vi "read_GPX_file.vi"(4 "error in":errorcluster, 7 "GPX File Path":path) -> (0 "error out":errorcluster, 1 "position Graph":cluster{"X":dbl, "Y":dbl}[](graph), 2 "lat/lon position":cluster{timestamp[], dbl[], dbl[]}, 3 "XY Speed data":cluster{timestamp[], dbl[]})   [LabVIEW 2020]
panel:
  out "trk.trkseg data":T1
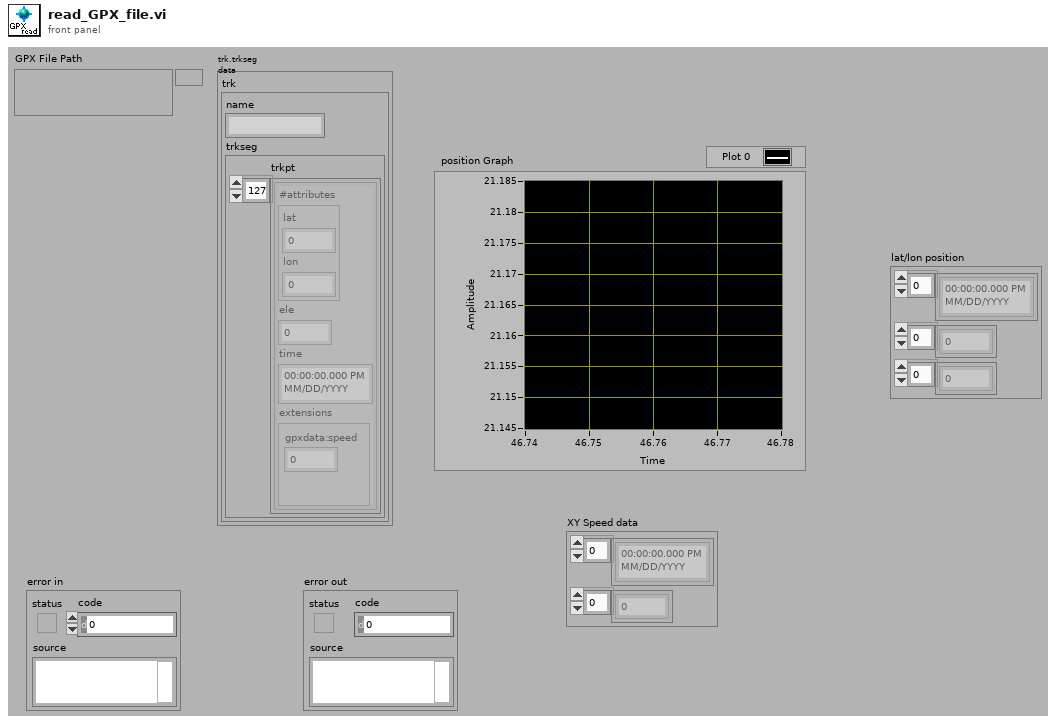
[diagram p1: front panel]
types:
  T1 = cluster{"trk":cluster{"name":string, "trkseg":cluster{"trkpt":cluster{"#attributes":cluster{"lat":dbl, "lon":dbl}, "ele":dbl, "time":timestamp, "extensions":cluster{"gpxdata:speed":dbl}}[]}}}
  T2 = cluster{"#attributes":cluster{"lat":dbl, "lon":dbl}, "ele":dbl, "time":timestamp, "extensions":cluster{"gpxdata:speed":dbl}}[]
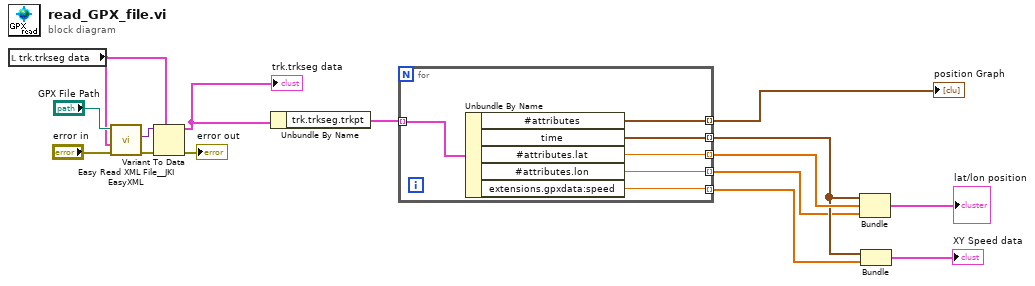
[diagram p0: block diagram]
diagram:
  n1 = local read "trk.trkseg data"() -> (w13:T1)
  n2 = call <vilib>:"Easy Read XML File__JKI EasyXML.vi"("error in (no error)"="error in", "LabVIEW Data (Type)"=w13, "XML File Path"="GPX File Path") -> ("error out"=w12:errorcluster, "LabVIEW Data"=w14:variant)  [unwired: 6 in, 1 out]
  n3 = Variant To Data(error in=w12, type=w13, Variant=w14) -> (data=w7:T1, error out=→"error out":errorcluster)
  "trk.trkseg data" <- w7
  n4 = Unbundle By Name(w7) -> ("trk.trkseg.trkpt"=w8:T2)
  n5 = for {
    tunnel: w8 -> [w21] mode=indexing
    tunnel: [w20] -> w9 mode=indexing
    tunnel: [w19] -> w4 mode=indexing
    tunnel: [w17] -> w5 mode=indexing
    tunnel: [w18] -> w2 mode=indexing
    tunnel: [w16] -> w3 mode=indexing
    n6 = Unbundle By Name(w21) -> ("#attributes"=w20:cluster{"lat":dbl, "lon":dbl}, "time"=w19:timestamp, "#attributes.lat"=w17:dbl, "#attributes.lon"=w18:dbl, "extensions.gpxdata:speed"=w16:dbl)
  }
  "position Graph" <- w9
  n7 = Bundle(w4, w5, w2) -> (→"lat/lon position":cluster{timestamp[], dbl[], dbl[]})  [unwired: 1 in]
  n8 = Bundle(w4, w3) -> (→"XY Speed data":cluster{timestamp[], dbl[]})  [unwired: 1 in]
